vi "GUID.vi"() -> (1 "error out":errorcluster, 2 "GUID":string)   [LabVIEW 2015]
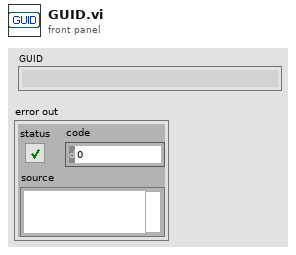
[diagram p1: front panel]
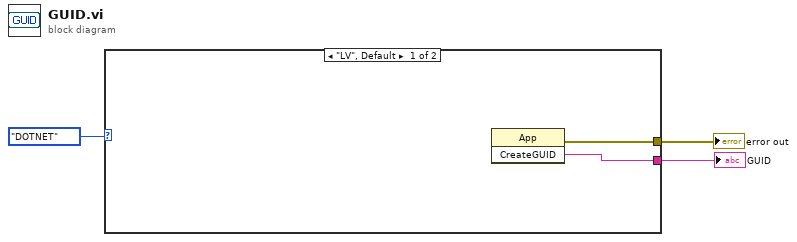
[diagram p0: block diagram]
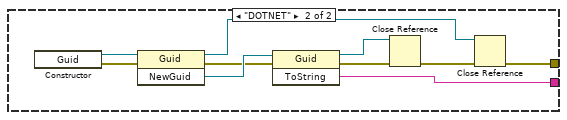
[diagram p2: hidden frame]
diagram:
  n1 = case shown="\"LV\", Default" enum16{"LV", "DOTNET"}."DOTNET" {
    tunnel: [w4 w7] -> w3
    tunnel: [w5 w6] -> w2
    frame "LV", Default {
      n2 = invoke class="App" method="CreateGUID"() -> (error out=w4:errorcluster, "CreateGUID"=w5:string)  [unwired: 3 in, 1 out]
    }
    frame "DOTNET" {
      n3 = constructor class="Guid"() -> (reference out=w15:refnum<k24>, error out=w14:errorcluster)  [unwired: 3 in, 1 out]
      n4 = invoke class="Guid" method="NewGuid"(reference=w15, error in=w14) -> (reference out=w8:refnum<k24>, error out=w12:errorcluster, "NewGuid"=w13:refnum<k24>)  [unwired: 1 in]
      n5 = invoke class="Guid" method="ToString"(reference=w13, error in=w12) -> (reference out=w10:refnum<k24>, error out=w11:errorcluster, "ToString"=w6:string)  [unwired: 1 in]
      n6 = Close Reference(reference=w10, error in (no error)=w11) -> (error out=w9:errorcluster)
      n7 = Close Reference(reference=w8, error in (no error)=w9) -> (error out=w7:errorcluster)
    }
  }
  "error out" <- w3
  "GUID" <- w2
